vi "Get Bus Enabled Properties.vi"(8 "error in (no error)":errorcluster, 11 "Item Ref in":T2 format="%.0x") -> (0 "error out":errorcluster, 2 "BusEnabledProperties":T1, 3 "Item Ref out":T2 format="%.0x")   [LabVIEW 2011, in "AIT 1553 Custom Device.lvlib"]
uses:
  AIT 1553 Custom Device.lvlib
  <vilib>/NI Veristand/Custom Device API/Custom Device Item Ref.ctl
  Controls/1553 Bus Enabled.ctl
  Controls and Global/Global.vi
  <vilib>/NI Veristand/Custom Device API/Get Item Property (Boolean).vi
  <vilib>/NI Veristand/Custom Device API/Custom Device API.lvlib
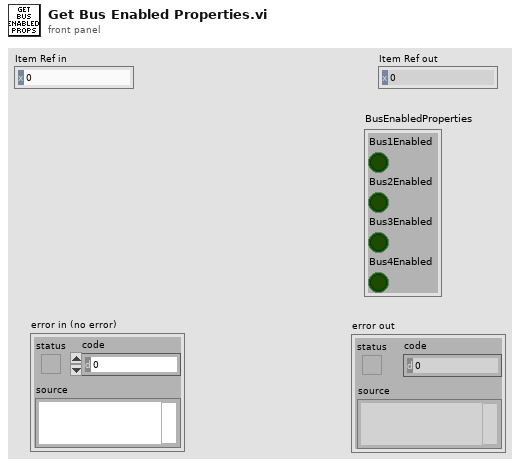
[diagram p1: front panel]
types:
  T1 = typedef "AIT 1553 Custom Device.lvlib/1553 Bus Enabled.ctl" = cluster{"Bus1Enabled":bool, "Bus2Enabled":bool, "Bus3Enabled":bool, "Bus4Enabled":bool}
  T2 = typedef "Custom Device API.lvlib/Custom Device Item Ref.ctl" = u64
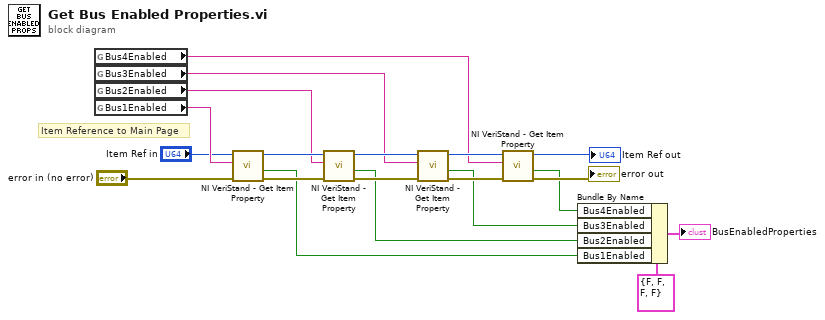
[diagram p0: block diagram]
diagram:
  # "Item Reference to Main Page"
  n1 = global read "Global.vi" "Bus4Enabled"() -> (w10:string)
  n2 = global read "Global.vi" "Bus3Enabled"() -> (w11:string)
  n3 = global read "Global.vi" "Bus2Enabled"() -> (w12:string)
  n4 = global read "Global.vi" "Bus1Enabled"() -> (w19:string)
  n5 = call-poly <vilib>:"NI VeriStand - Get Item Property.vi"("error in (no error)"="error in (no error)", "Property Name"=w19, "Item Ref in"="Item Ref in") -> ("error out"=w15:errorcluster, "Value"=w5:bool, "Item Ref out"=w18:T2)  [unwired: 5 in, 1 out]
  n6 = call-poly <vilib>:"NI VeriStand - Get Item Property.vi"("error in (no error)"=w15, "Property Name"=w12, "Item Ref in"=w18) -> ("error out"=w14:errorcluster, "Value"=w4:bool, "Item Ref out"=w17:T2)  [unwired: 5 in, 1 out]
  n7 = call-poly <vilib>:"NI VeriStand - Get Item Property.vi"("error in (no error)"=w14, "Property Name"=w11, "Item Ref in"=w17) -> ("error out"=w13:errorcluster, "Value"=w3:bool, "Item Ref out"=w16:T2)  [unwired: 5 in, 1 out]
  n8 = call-poly <vilib>:"NI VeriStand - Get Item Property.vi"("error in (no error)"=w13, "Property Name"=w10, "Item Ref in"=w16) -> ("error out"=→"error out":errorcluster, "Value"=w2:bool, "Item Ref out"=→"Item Ref out":T2)  [unwired: 5 in, 1 out]
  n9 = Bundle By Name(cluster=T1 {"Bus1Enabled"=FALSE, "Bus2Enabled"=FALSE, "Bus3Enabled"=FALSE, "Bus4Enabled"=FALSE} ("BusEnabledProperties"), "Bus4Enabled"=w2, "Bus3Enabled"=w3, "Bus2Enabled"=w4, "Bus1Enabled"=w5) -> (→"BusEnabledProperties":T1)
